vi "Turret Align.vi"() -> ()   [LabVIEW 2019]
panel:
  out "Meter":dbl(knob) scale=-30.0..30.0
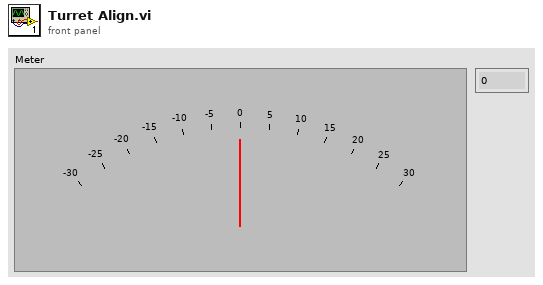
[diagram p1: front panel]
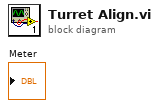
[diagram p0: block diagram]
diagram:
